vi "Nominal Frequency.vi"(11 "Master Controller in":refnum<class "EMS User Interface.lvclass">) -> ()   [LabVIEW 2018, in "EMS User Interface Actor.lvlib" / "EMS User Interface.lvclass"]
uses:
  EMS User Interface.lvclass
  C:/Users/Administrator/Desktop/LabVIEW EMS/EMS Generic Actor/EMS Generic/EMS Generic.lvclass
  C:/Program Files (x86)/National Instruments/LabVIEW 2018/vi.lib/ActorFramework/Actor/Actor.lvclass
  <vilib>/ActorFramework/Actor/Actor.lvclass/Actor.ctl
  <vilib>/ActorFramework/Message Enqueuer/Message Enqueuer.lvclass/Message Enqueuer.ctl
  EMS User Interface Messages/Write Nominal Frequency Msg/Write Nominal Frequency Msg.lvclass/Write Nominal Frequency Msg.ctl
  <vilib>/ActorFramework/Message Enqueuer/Init from Existing Queue.vi
  <vilib>/ActorFramework/Message Enqueuer/Enqueue.vi
  EMS User Interface Messages/Write Nominal Frequency Msg/Write Nominal Frequency Msg.lvclass
  C:/Program Files (x86)/National Instruments/LabVIEW 2018/vi.lib/ActorFramework/Message/Message.lvclass
  <vilib>/ActorFramework/Message Priority Queue/Priority Enqueue.vi
  <vilib>/ActorFramework/Message Enqueuer/Message Enqueuer.lvclass
  <vilib>/ActorFramework/Actor/Actor.lvclass
  EMS Generic Actor/EMS Generic/EMS Generic.lvclass
panel:
  in  "error in":errorcluster
  in  "Cancel":bool
  in  "OK":bool
  in  "Numeric":dbl
  # "Specify Nominal Frequency"
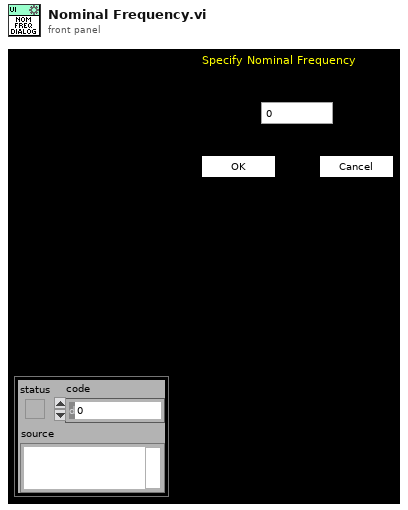
[diagram p1: front panel]
types:
  T1 = enum32{"Invalid", "Standard", "Closed", "Hidden", "Minimized", "Maximized"}
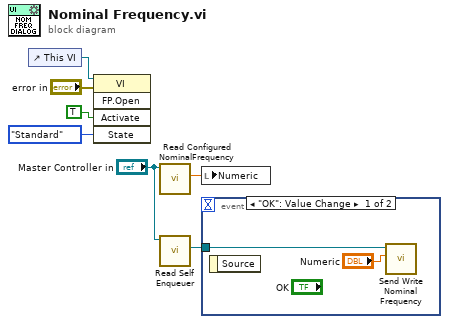
[diagram p0: block diagram]
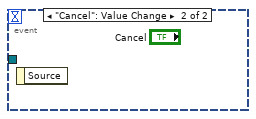
[diagram p2: hidden frame]
diagram:
  n1 = control-ref of="This VI"() -> (w6:refnum<vi>)
  n2 = invoke class="VI" method="FP.Open"(reference=w6, error in="error in", "Activate"=TRUE ("Activate?"), "State"=T1."Standard") -> ()  [unwired: 1 in, 5 out]
  n3 = call "Read Configured NominalFrequency.vi"("EMS Generic in"="Master Controller in") -> ("NominalFrequency"=w1:dbl)  [unwired: 8 in, 2 out]
  n4 = call <vilib>:"Read Self Enqueuer.vi"("Actor"="Master Controller in") -> ("Self Enqueuer"=w7:refnum<class "Message Enqueuer.lvclass">)  [unwired: 10 in]
  n5 = local write "Numeric"(w1) -> ()
  n6 = event shown="[0] \"OK\": Value Change" {
    selector: _ -> [_ _]
    dyn-events: _ -> [_ _]
    timeout: _ -> [_ _]
    tunnel: w7 -> [w9 _]
    event "OK": Value Change {
      n7 = event-data() -> ()  [unwired: 1 in, 1 out]
      n8 = call "Send Write Nominal Frequency.vi"("Nominal Frequency"="Numeric", "Message Enqueuer"=w9) -> ()  [unwired: 8 in, 2 out]
    }
    event "Cancel": Value Change {
      n9 = event-data() -> ()  [unwired: 1 in, 1 out]
    }
  }
